vi "Production_of_Baker'sYeast_Repetitive_Fed_batch.vi"() -> ()   [LabVIEW 2019]
uses:
  <vilib>/addons/control/pid/pid.llb/PID Advanced (DBL).vi
  <vilib>/addons/control/pid/NI_PID_pid.lvlib
panel:
  out "Glucose Pipe 2":bool
  in  "process parameters":T1={"static gain"=2.5, "lag (s)"=2.5, "deadtime (s)"=0.001, "load"=0.0, "deadband"=0.0, "sensor noise"=0.0, "initial PV"=30.0, "plant noise"=0.0} {"plant noise" format="%.2f"; "initial PV" format="%.2f"; "sensor noise" format="%.2f"; "lag (s)" format="%.2f"; "deadtime (s)" format="%.2f"; "deadband" format="%.1f"; "load" format="%.2f"; "static gain" format="%.2f"}
  in  "SP Glucose 2":dbl(slide) scale=0.0..10.0
  in  "SP":dbl(knob) scale=0.0..100.0
  in  "auto? (T) 2":bool=TRUE
  in  "PID gains 2":T2={"proportional gain (Kc)"=1.0, "integral time (Ti, min)"=0.01, "derivative time (Td, min)"=0.0} {"derivative time (Td, min)" format="%.3f"; "integral time (Ti, min)" format="%.3f"; "proportional gain (Kc)" format="%.3f"}
  in  "LCV 2":dbl format="%.2f"
  out "Waveform Chart 2":T3(graph)
  out "Thermometer":dbl(slide) scale=0.0..100.0
  in  "process parameters 2":T1={"static gain"=2.5, "lag (s)"=2.5, "deadtime (s)"=0.001, "load"=0.0, "deadband"=0.0, "sensor noise"=0.0, "initial PV"=30.0, "plant noise"=0.0} {"plant noise" format="%.2f"; "initial PV" format="%.2f"; "sensor noise" format="%.2f"; "lag (s)" format="%.2f"; "deadtime (s)" format="%.2f"; "deadband" format="%.1f"; "load" format="%.2f"; "static gain" format="%.2f"}
  in  "LCV":dbl format="%.2f"
  in  "auto? (T)":bool=TRUE
  in  "SP Glucose":dbl(slide) scale=0.0..10.0
  in  "PID gains":T2={"proportional gain (Kc)"=1.0, "integral time (Ti, min)"=0.01, "derivative time (Td, min)"=0.0} {"derivative time (Td, min)" format="%.3f"; "integral time (Ti, min)" format="%.3f"; "proportional gain (Kc)" format="%.3f"}
  out "Waveform Chart":cluster{"output":dbl, dbl, "Plant Output":dbl}(graph)
  out "Multi-Segment Pipe":bool(c317)
  out "Storage":i32(slide) scale=0.0..450.0
  out "GLUCOSE":dbl(slide) scale=0.0..100.0
  out "Yeast bool":bool
  out "Yeast Pipe":bool
  out "YEAST (saccharomyces cerevisiae)":dbl(slide) scale=0.0..100.0
  out "Gauge":dbl(knob) scale=0.0..100.0 scale format="%#_3g"
  out "MIddle  bool":bool
  out "middle pipe":bool
  out "reactor bool":bool
  out "Glucose bool":bool
  out "Glucose Pipe":bool
  out "Mixtures":i32(slide) scale=0.0..250.0
  # "LCV"
  # "LT"
  # "REACTOR"
  # "CONTROL ROOM"
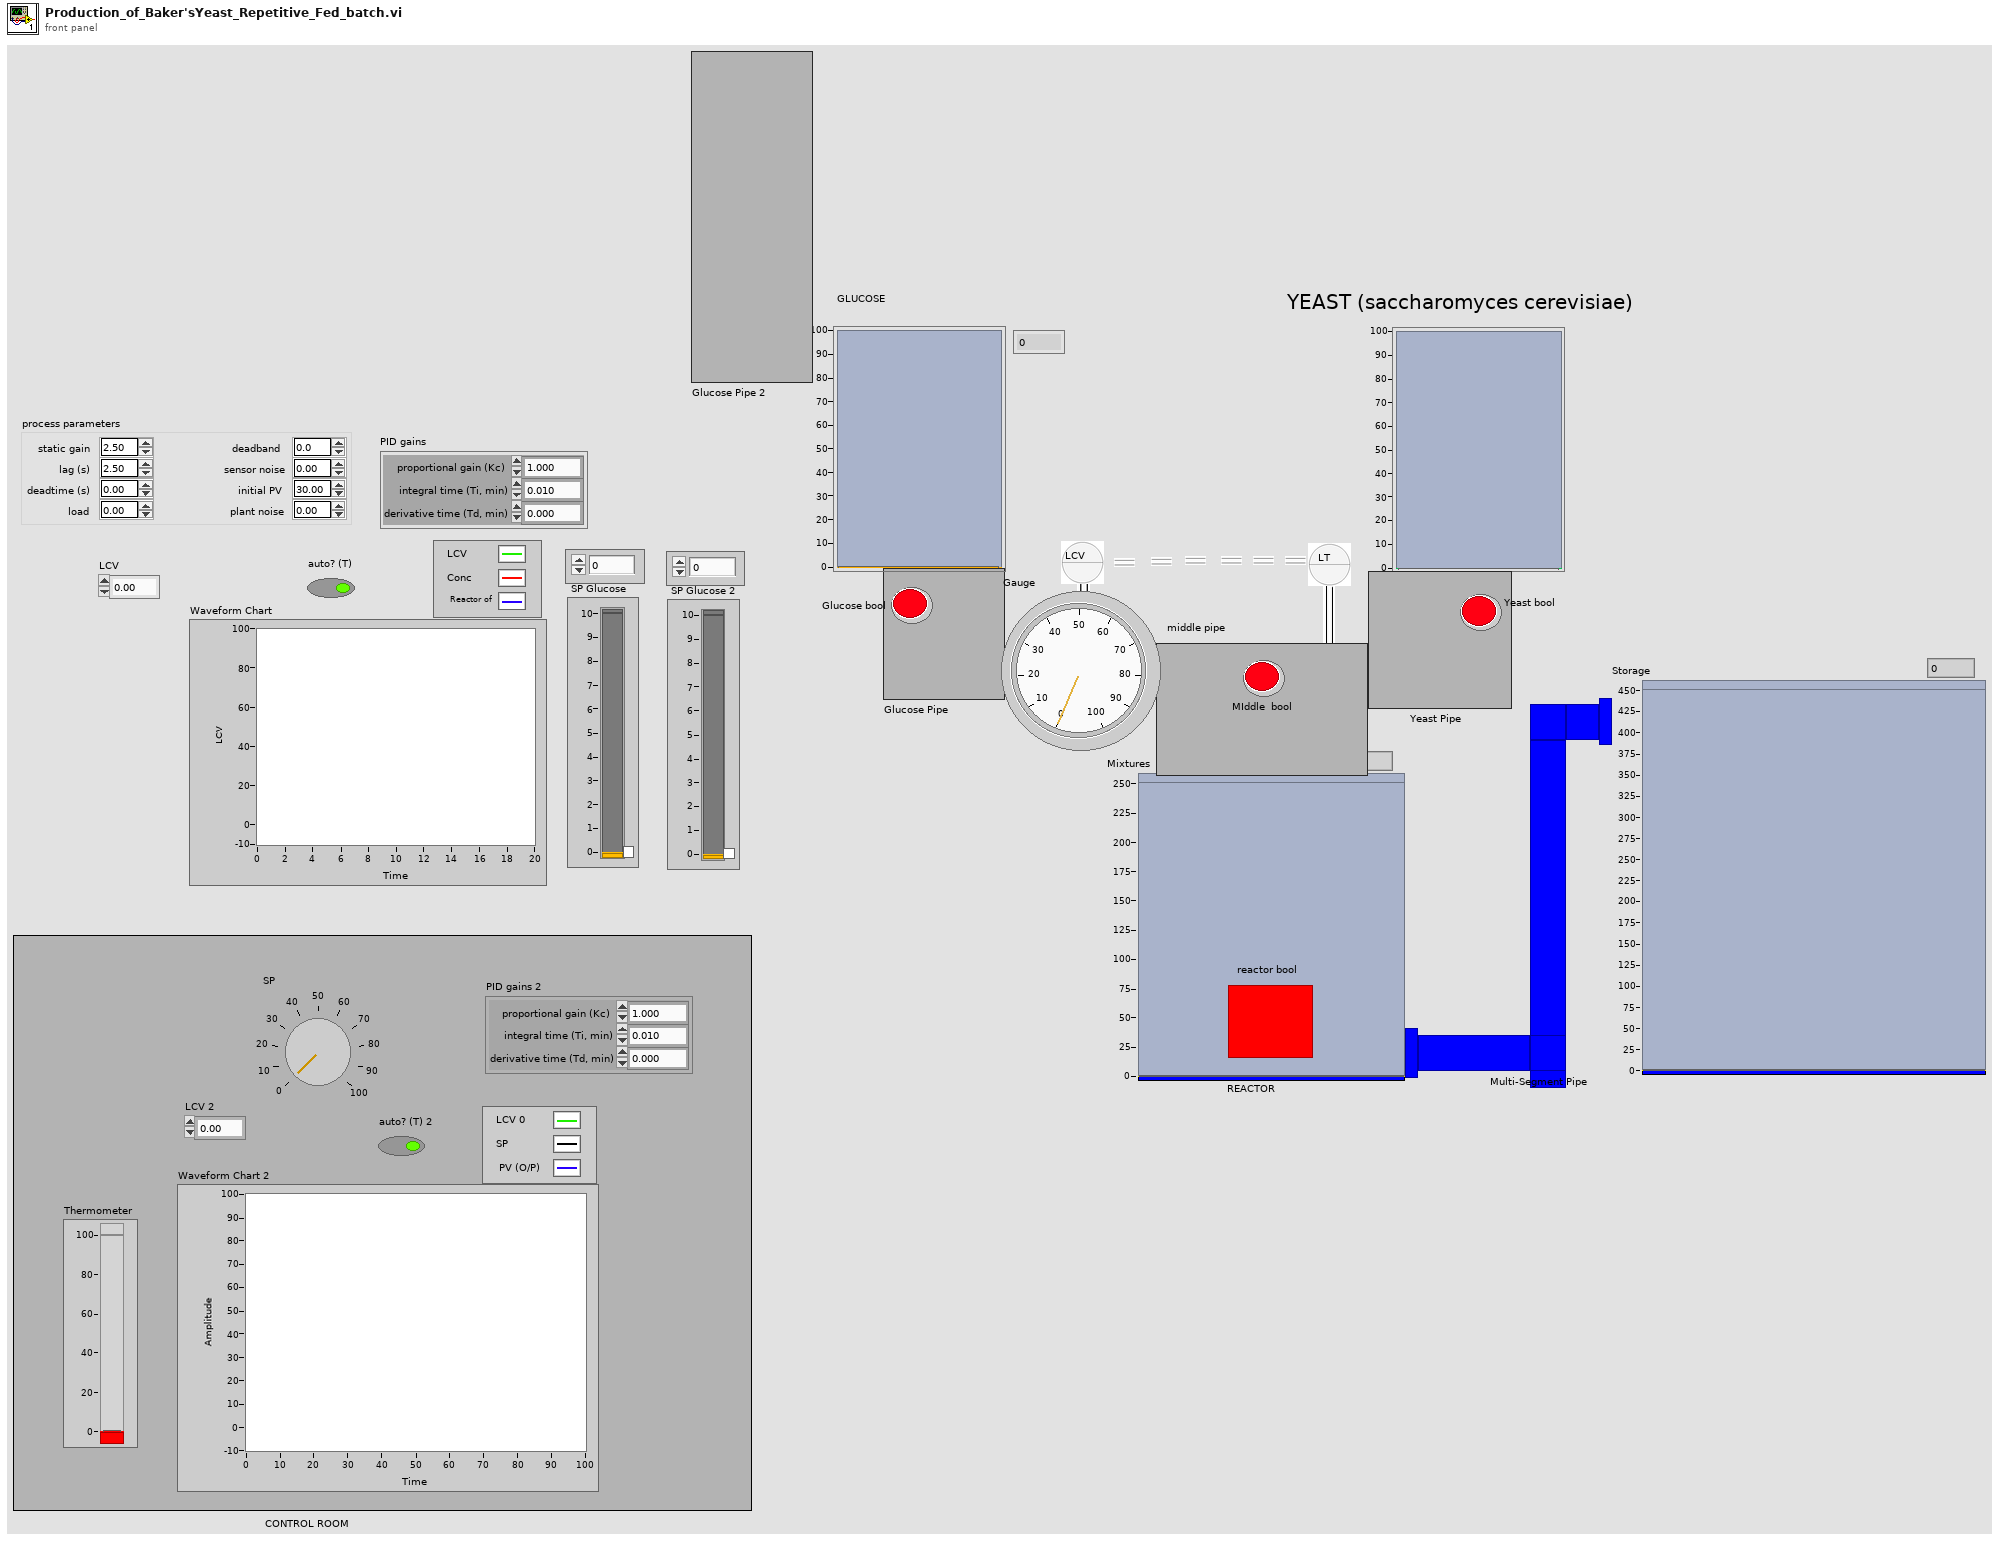
[diagram p1: front panel]
types:
  T1 = cluster{"static gain":dbl, "lag (s)":dbl, "deadtime (s)":dbl, "load":dbl, "deadband":dbl, "sensor noise":dbl, "initial PV":dbl, "plant noise":dbl}
  T2 = cluster{"proportional gain (Kc)":dbl, "integral time (Ti, min)":dbl, "derivative time (Td, min)":dbl}
  T3 = cluster{"LCV":dbl, " SP":dbl, "Plant Output":dbl}
  T4 = cluster{"output":dbl, "SP":dbl, "Plant Output":dbl}
diagram:
  n1 = flat-sequence {
    frame #0 {
      n2 = while {
        shift-right: [w17] -> _
        shift-left: 30.0 -> [w15]
        tunnel: TRUE ("Yeast bool") -> [w11]
        tunnel: FALSE ("Glucose bool") -> [w10]
        tunnel: FALSE ("reactor bool") -> [w9]
        tunnel: 0.0 ("Gauge") -> [w7]
        tunnel: 30.0 ("GLUCOSE") -> [w8]
        stop <- w13 stop-if-true
        n3 = property on="Storage" class="Slide (strict)"("Value"=w7) -> ()  [unwired: 2 in, 2 out]
        n4 = property on="Gauge" class="Knob (strict)"("Value"=w7) -> ()  [unwired: 2 in, 2 out]
        n5 = property on="GLUCOSE" class="Slide (strict)"("Value"=w8) -> ()  [unwired: 2 in, 2 out]
        n6 = property on="reactor bool" class="Bool (strict)"("Value"=w9) -> ()  [unwired: 2 in, 2 out]
        n7 = property on="MIddle  bool" class="Bool (strict)"("Value"=w11) -> ()  [unwired: 2 in, 2 out]
        n8 = property on="Glucose bool" class="Bool (strict)"("Value"=w10) -> ()  [unwired: 2 in, 2 out]
        n9 = Wait Until Next ms Multiple(millisecond multiple=u32 400) -> ()  [unwired: 1 out]
        n10 = property on="middle pipe" class="Bool (strict)"("Value"=w11) -> ()  [unwired: 2 in, 2 out]
        n11 = property on="Glucose Pipe" class="Bool (strict)"("Value"=w10) -> ()  [unwired: 2 in, 2 out]
        n12 = Subtract(x=30.0, y=w15) -> (x-y=w12:dbl)
        n13 = Equal?(x=w15, y=0.0) -> (x = y?=w13:bool)
        n14 = Decrement(x=w15) -> (x-1=w17:dbl)
        n15 = property on="Mixtures" class="Slide (strict)"("Value"=w12) -> ()  [unwired: 2 in, 2 out]
        "YEAST (saccharomyces cerevisiae)" <- w15
        "Yeast Pipe" <- w11
        "Yeast bool" <- w11
      }
    }
    frame #1 {
      n16 = while {
        border: 0.0 ("Plant Output") -> [_]
        tunnel: FALSE ("reactor bool") -> [w50]
        tunnel: TRUE ("Glucose bool") -> [w54]
        tunnel: TRUE ("MIddle  bool") -> [w53]
        stop <- w30 stop-if-true
        w38 = u32 100 ("millisecond multiple")
        w65 = u32 100 ("millisecond multiple")
        n17 = property on="Yeast bool" class="Bool (strict)"("Value"=w50) -> ()  [unwired: 2 in, 2 out]
        n18 = property on="reactor bool" class="Bool (strict)"("Value"=w50) -> ()  [unwired: 2 in, 2 out]
        n19 = property on="Yeast Pipe" class="Bool (strict)"("Value"=w50) -> ()  [unwired: 2 in, 2 out]
        n20 = Wait Until Next ms Multiple(millisecond multiple=w65) -> ()  [unwired: 1 out]
        n21 = Multiply(x=0.001, y=w65) -> (x*y=w40:dbl)
        n22 = Add(x="SP Glucose", y=30.0) -> (x+y=w49:dbl)
        n23 = Wait Until Next ms Multiple(millisecond multiple=w38) -> ()  [unwired: 1 out]
        n24 = Multiply(x=0.001, y=w38) -> (x*y=w36:dbl)
        n25 = property on="SP Glucose" class="Slide (strict)"() -> ("Value"=w26:dbl)  [unwired: 2 in, 2 out]
        n26 = Subtract(x=30.0 ("y"), y=w26) -> (x-y=w45:dbl)
        n27 = Wait Until Next ms Multiple(millisecond multiple=u32 600) -> ()  [unwired: 1 out]
        n28 = feedback #1() -> (w64:dbl)
        n29 = call-poly <vilib>:"PID Advanced.vi"("setpoint"=w49, "output range"=cluster{"output high":dbl, "output low":dbl} {"output high"=100.0, "output low"=0.0}, "auto? (T)"="auto? (T)", "manual control"="LCV", "process variable"=w64, "PID gains"="PID gains", "dt (s)"=w40) -> ("output"=w47:dbl)  [unwired: 7 in, 1 out]
        "Gauge" <- w47
        n30 = feedback #2() -> (w35:dbl)  [unwired: 1 in]
        n31 = call-poly <vilib>:"PID Advanced.vi"("setpoint"=w45, "output range"=cluster{"output high":dbl, "output low":dbl} {"output high"=100.0, "output low"=0.0}, "auto? (T)"="auto? (T)", "manual control"="LCV", "process variable"=w35, "PID gains"="PID gains", "dt (s)"=w36) -> ("output"=w24:dbl)  [unwired: 7 in, 1 out]
        n32 = property on="process parameters" class="Clust (strict)"() -> ("Value"=w23:T1)  [unwired: 2 in, 2 out]
        n33 = call "Plant System.vi"("output saturation range"=cluster{"output high":dbl, "output low":dbl} {"output high"=100.0, "output low"=0.0}, "Plant Input"=w47, "dt (s)"=w40, "process parameters"=w23) -> ("Plant Output"=w46:dbl)  [unwired: 11 in]
        n34 = feedback-in #1(w46) -> ()
        n35 = call "Plant System.vi"("output saturation range"=cluster{"output high":dbl, "output low":dbl} {"output high"=100.0, "output low"=0.0}, "Plant Input"=w24, "dt (s)"=w36, "process parameters"=w23) -> ("Plant Output"=w34:dbl)  [unwired: 11 in]
        "GLUCOSE" <- w34
        n36 = feedback-in #2(w34) -> ()
        n37 = property on="SP Glucose" class="Slide (strict)"() -> ("Value"=w59:dbl)  [unwired: 2 in, 2 out]
        n38 = property on="SP Glucose" class="Slide (strict)"() -> ("Value"=w29:dbl)  [unwired: 2 in, 2 out]
        n39 = Bundle("output"=w47, w49, "Plant Output"=w46) -> (→"Waveform Chart":cluster{"output":dbl, dbl, "Plant Output":dbl})  [unwired: 1 in]
        n40 = Add(x=30.0, y=w59) -> (x+y=w58:dbl)
        n41 = property on="Mixtures" class="Slide (strict)"() -> ("Value"=w52:i32)  [unwired: 2 in, 2 out]
        n42 = property on="GLUCOSE" class="Slide (strict)"() -> ("Value"=w33:dbl)  [unwired: 2 in, 2 out]
        n43 = Subtract(x=30.0, y=w29) -> (x-y=w25:dbl)
        n44 = Add(x=w46, y=0.0) -> (x+y=→"Mixtures":dbl)
        n45 = Greater Or Equal?(x=w52, y=w58) -> (x >= y?=w32:bool)
        n46 = Less Or Equal?(x=w33, y=w25) -> (x <= y?=w31:bool)
        n47 = And(x=w32, y=w31) -> (x .and. y?=w30:bool)
        "Glucose bool" <- w54
        "Glucose Pipe" <- w54
        "MIddle  bool" <- w53
        "middle pipe" <- w53
      }
    }
    frame #2 {
      n48 = while {
        stop <- w67 stop-if-true
        w80 = u32 100 ("millisecond multiple")
        n49 = Wait Until Next ms Multiple(millisecond multiple=w80) -> ()  [unwired: 1 out]
        n50 = Multiply(x=0.001, y=w80) -> (x*y=w78:dbl)
        n51 = property on="Thermometer" class="Slide (strict)"() -> ("Value"=w70:dbl)  [unwired: 2 in, 2 out]
        n52 = call-poly <vilib>:"PID Advanced.vi"("setpoint"="SP", "output range"=cluster{"output high":dbl, "output low":dbl} {"output high"=100.0, "output low"=0.0}, "auto? (T)"="auto? (T) 2", "manual control"="LCV 2", "process variable"=w70, "PID gains"="PID gains 2", "dt (s)"=w78) -> ("output"=w74:dbl)  [unwired: 7 in, 1 out]
        n53 = call "Plant System.vi"("output saturation range"=cluster{"output high":dbl, "output low":dbl} {"output high"=100.0, "output low"=0.0}, "Plant Input"=w74, "dt (s)"=w78, "process parameters"="process parameters 2") -> ("Plant Output"=w72:dbl)  [unwired: 11 in]
        "Thermometer" <- w72
        n54 = Bundle("output"=w74, "SP"="SP", "Plant Output"=w72) -> (→"Waveform Chart 2":T4)  [unwired: 1 in]
        n55 = property on="Thermometer" class="Slide (strict)"() -> ("Value"=w69:dbl)  [unwired: 2 in, 2 out]
        n56 = property on="SP" class="Knob (strict)"() -> ("Value"=w68:dbl)  [unwired: 2 in, 2 out]
        n57 = Greater Or Equal?(x=w69, y=w68) -> (x >= y?=w67:bool)
      }
    }
    frame #3 {
      n58 = property on="Mixtures" class="Slide (strict)"() -> ("Value"=w85:i32)  [unwired: 2 in, 2 out]
      n59 = while {
        shift-right: [w93] -> _
        shift-left: w85 -> [w94]
        tunnel: TRUE ("reactor bool") -> [w92]
        stop <- w95 stop-if-true
        n60 = property on="SP Glucose" class="Slide (strict)"() -> ("Value"=w87:dbl)  [unwired: 2 in, 2 out]
        n61 = Add(x=30.0, y=w87) -> (x+y=w86:dbl)
        n62 = property on="Mixtures" class="Slide (strict)"("Value"=w94) -> ()  [unwired: 2 in, 2 out]
        n63 = Scale By Power Of 2(n=i16 2, x=w86) -> (x*2^n=w89:dbl)
        n64 = Increment(x=w94) -> (x+1=w93:i32)
        n65 = Greater Or Equal?(x=w93, y=w89) -> (x >= y?=w95:bool)
        n66 = Wait Until Next ms Multiple(millisecond multiple=u32 1000) -> ()  [unwired: 1 out]
        "reactor bool" <- w92
      }
    }
    frame #4 {
      n67 = property on="Mixtures" class="Slide (strict)"() -> ("Value"=w97:i32)  [unwired: 2 in, 2 out]
      n68 = while {
        shift-right: [w110] -> _
        shift-left: w97 -> [w106]
        tunnel: TRUE ("Multi-Segment Pipe") -> [w104]
        stop <- w108 stop-if-true
        n69 = property on="SP Glucose" class="Slide (strict)"() -> ("Value"=w99:dbl)  [unwired: 2 in, 2 out]
        n70 = Wait Until Next ms Multiple(millisecond multiple=u32 400) -> ()  [unwired: 1 out]
        n71 = Add(x=30.0, y=w99) -> (x+y=w98:dbl)
        n72 = property on="Mixtures" class="Slide (strict)"("Value"=w106) -> ()  [unwired: 2 in, 2 out]
        n73 = Scale By Power Of 2(n=i16 2, x=w98) -> (x*2^n=w102:dbl)
        n74 = Add(x=0.0, y=w102) -> (x+y=w105:dbl)
        n75 = Equal?(x=w106, y=30.0) -> (x = y?=w108:bool)
        n76 = Subtract(x=w105, y=w106) -> (x-y=→"Storage":dbl)
        n77 = Decrement(x=w106) -> (x-1=w110:i32)
        "Multi-Segment Pipe" <- w104
      }
    }
    frame #5 {
      n78 = property on="GLUCOSE" class="Slide (strict)"() -> ("Value"=w114:dbl)  [unwired: 2 in, 2 out]
      n79 = while {
        shift-right: [w120] -> _
        shift-left: w114 -> [w118]
        tunnel: TRUE ("Glucose Pipe 2") -> [w116]
        tunnel: TRUE ("reactor bool") -> [w115]
        stop <- w121 stop-if-true
        n80 = property on="reactor bool" class="Bool (strict)"("Value"=w115) -> ()  [unwired: 2 in, 2 out]
        n81 = property on="GLUCOSE" class="Slide (strict)"("Value"=w118) -> ()  [unwired: 2 in, 2 out]
        n82 = Increment(x=w118) -> (x+1=w120:dbl)
        n83 = Greater Or Equal?(x=w120, y=30.0) -> (x >= y?=w121:bool)
        n84 = Wait Until Next ms Multiple(millisecond multiple=u32 1000) -> ()  [unwired: 1 out]
        "Glucose Pipe 2" <- w116
      }
    }
    frame #6 {
      n85 = while {
        border: 0.0 ("Plant Output") -> [_]
        tunnel: FALSE ("reactor bool") -> [w127]
        tunnel: TRUE ("Glucose bool") -> [w134]
        tunnel: TRUE ("MIddle  bool") -> [w126]
        stop <- w150 stop-if-true
        w156 = u32 100 ("millisecond multiple")
        w170 = u32 100 ("millisecond multiple")
        n86 = property on="reactor bool" class="Bool (strict)"("Value"=w126) -> ()  [unwired: 2 in, 2 out]
        n87 = property on="middle pipe" class="Bool (strict)"("Value"=w126) -> ()  [unwired: 2 in, 2 out]
        n88 = property on="Glucose Pipe" class="Bool (strict)"("Value"=w126) -> ()  [unwired: 2 in, 2 out]
        n89 = property on="Yeast bool" class="Bool (strict)"("Value"=w127) -> ()  [unwired: 2 in, 2 out]
        n90 = property on="MIddle  bool" class="Bool (strict)"("Value"=w134) -> ()  [unwired: 2 in, 2 out]
        n91 = property on="PID gains" class="Clust (strict)"() -> ("Value"=w146:T2)  [unwired: 2 in, 2 out]
        n92 = property on="Yeast Pipe" class="Bool (strict)"("Value"=w127) -> ()  [unwired: 2 in, 2 out]
        n93 = property on="Glucose bool" class="Bool (strict)"("Value"=w134) -> ()  [unwired: 2 in, 2 out]
        n94 = Wait Until Next ms Multiple(millisecond multiple=w170) -> ()  [unwired: 1 out]
        n95 = Multiply(x=0.001, y=w170) -> (x*y=w158:dbl)
        n96 = property on="SP Glucose 2" class="Slide (strict)"() -> ("Value"=w130:dbl)  [unwired: 2 in, 2 out]
        n97 = property on="LCV" class="DigNum (strict)"() -> ("Value"=w144:dbl)  [unwired: 2 in, 2 out]
        n98 = Add(x="SP Glucose 2", y=30.0) -> (x+y=w163:dbl)
        n99 = property on="auto? (T)" class="Bool (strict)"() -> ("Value"=w145:bool)  [unwired: 2 in, 2 out]
        n100 = Wait Until Next ms Multiple(millisecond multiple=w156) -> ()  [unwired: 1 out]
        n101 = Multiply(x=0.001, y=w156) -> (x*y=w154:dbl)
        n102 = Subtract(x=30.0, y=w130) -> (x-y=w132:dbl)
        n103 = Subtract(x=0.0, y=w132) -> (x-y=w160:dbl)
        n104 = Wait Until Next ms Multiple(millisecond multiple=u32 600) -> ()  [unwired: 1 out]
        n105 = feedback #3() -> (w169:dbl)
        n106 = call-poly <vilib>:"PID Advanced.vi"("setpoint"=w163, "output range"=cluster{"output high":dbl, "output low":dbl} {"output high"=100.0, "output low"=0.0}, "auto? (T)"=w145, "manual control"=w144, "process variable"=w169, "PID gains"=w146, "dt (s)"=w158) -> ("output"=w135:dbl)  [unwired: 7 in, 1 out]
        n107 = feedback #4() -> (w153:dbl)  [unwired: 1 in]
        n108 = call-poly <vilib>:"PID Advanced.vi"("setpoint"=w160, "output range"=cluster{"output high":dbl, "output low":dbl} {"output high"=100.0, "output low"=0.0}, "auto? (T)"=w145, "manual control"=w144, "process variable"=w153, "PID gains"=w146, "dt (s)"=w154) -> ("output"=w147:dbl)  [unwired: 7 in, 1 out]
        n109 = call "Plant System.vi"("output saturation range"=cluster{"output high":dbl, "output low":dbl} {"output high"=100.0, "output low"=0.0}, "Plant Input"=w135, "dt (s)"=w158, "process parameters"="process parameters") -> ("Plant Output"=w161:dbl)  [unwired: 11 in]
        n110 = feedback-in #3(w161) -> ()
        n111 = call "Plant System.vi"("output saturation range"=cluster{"output high":dbl, "output low":dbl} {"output high"=100.0, "output low"=0.0}, "Plant Input"=w147, "dt (s)"=w154, "process parameters"="process parameters") -> ("Plant Output"=w136:dbl)  [unwired: 11 in]
        n112 = feedback-in #4(w136) -> ()
        n113 = property on="Gauge" class="Knob (strict)"("Value"=w135) -> ()  [unwired: 2 in, 2 out]
        n114 = property on="SP Glucose 2" class="Slide (strict)"() -> ("Value"=w139:dbl)  [unwired: 2 in, 2 out]
        n115 = property on="SP Glucose 2" class="Slide (strict)"() -> ("Value"=w137:dbl)  [unwired: 2 in, 2 out]
        n116 = Bundle("output"=w135, w163, "Plant Output"=w161) -> (w142:cluster{"output":dbl, dbl, "Plant Output":dbl})  [unwired: 1 in]
        n117 = property on="Mixtures" class="Slide (strict)"() -> ("Value"=w138:i32)  [unwired: 2 in, 2 out]
        n118 = property on="GLUCOSE" class="Slide (strict)"() -> ("Value"=w143:dbl)  [unwired: 2 in, 2 out]
        n119 = Add(x=30.0, y=w139) -> (x+y=w166:dbl)
        n120 = Subtract(x=30.0, y=w137) -> (x-y=w148:dbl)
        n121 = Add(x=w161, y=0.0) -> (x+y=w141:dbl)
        n122 = Greater Or Equal?(x=w138, y=w166) -> (x >= y?=w152:bool)
        n123 = Less Or Equal?(x=w143, y=w148) -> (x <= y?=w151:bool)
        n124 = property on="Waveform Chart" class="WFChart (strict)"("Value"=w142) -> ()  [unwired: 2 in, 2 out]
        n125 = And(x=w152, y=w151) -> (x .and. y?=w150:bool)
        n126 = property on="Mixtures" class="Slide (strict)"("Value"=w141) -> ()  [unwired: 2 in, 2 out]
        n127 = property on="GLUCOSE" class="Slide (strict)"("Value"=w136) -> ()  [unwired: 2 in, 2 out]
      }
    }
    frame #7 {
      n128 = property on="Mixtures" class="Slide (strict)"() -> ("Value"=w174:i32)  [unwired: 2 in, 2 out]
      n129 = while {
        shift-right: [w184] -> _
        shift-left: w174 -> [w178]
        tunnel: TRUE ("reactor bool") -> [w176]
        tunnel: FALSE ("Glucose bool") -> [w175]
        stop <- w185 stop-if-true
        n130 = property on="SP Glucose 2" class="Slide (strict)"() -> ("Value"=w177:dbl)  [unwired: 2 in, 2 out]
        n131 = property on="Glucose bool" class="Bool (strict)"("Value"=w175) -> ()  [unwired: 2 in, 2 out]
        n132 = property on="reactor bool" class="Bool (strict)"("Value"=w176) -> ()  [unwired: 2 in, 2 out]
        n133 = Add(x=30.0, y=w177) -> (x+y=w179:dbl)
        n134 = property on="Mixtures" class="Slide (strict)"("Value"=w178) -> ()  [unwired: 2 in, 2 out]
        n135 = Scale By Power Of 2(n=i16 2, x=w179) -> (x*2^n=w181:dbl)
        n136 = property on="MIddle  bool" class="Bool (strict)"("Value"=w175) -> ()  [unwired: 2 in, 2 out]
        n137 = property on="Glucose Pipe" class="Bool (strict)"("Value"=w175) -> ()  [unwired: 2 in, 2 out]
        n138 = property on="middle pipe" class="Bool (strict)"("Value"=w175) -> ()  [unwired: 2 in, 2 out]
        n139 = Increment(x=w178) -> (x+1=w184:i32)
        n140 = Greater Or Equal?(x=w184, y=w181) -> (x >= y?=w185:bool)
        n141 = Wait Until Next ms Multiple(millisecond multiple=u32 1000) -> ()  [unwired: 1 out]
      }
    }
    frame #8 {
      n142 = property on="Mixtures" class="Slide (strict)"() -> ("Value"=w187:i32)  [unwired: 2 in, 2 out]
      n143 = while {
        shift-right: [w204] -> _
        shift-left: w187 -> [w196]
        tunnel: TRUE ("Multi-Segment Pipe") -> [w194]
        stop <- w202 stop-if-true
        n144 = property on="SP Glucose 2" class="Slide (strict)"() -> ("Value"=w195:dbl)  [unwired: 2 in, 2 out]
        n145 = property on="Multi-Segment Pipe" class="MultiSegPipe"("Value"=w194) -> ()  [unwired: 2 in, 2 out]
        n146 = Add(x=30.0, y=w195) -> (x+y=w193:dbl)
        n147 = Wait Until Next ms Multiple(millisecond multiple=u32 400) -> ()  [unwired: 1 out]
        n148 = Add(x=w193, y=0.0) -> (x+y=w192:dbl)
        n149 = property on="Mixtures" class="Slide (strict)"("Value"=w196) -> ()  [unwired: 2 in, 2 out]
        n150 = Scale By Power Of 2(n=i16 2, x=w192) -> (x*2^n=w199:dbl)
        n151 = Add(x=0.0, y=w199) -> (x+y=w201:dbl)
        n152 = Equal?(x=w196, y=0.0) -> (x = y?=w202:bool)
        n153 = Subtract(x=w201, y=w196) -> (x-y=w190:dbl)
        n154 = Decrement(x=w196) -> (x-1=w204:i32)
        n155 = Add(x=w190, y=110.0) -> (x+y=w191:dbl)
        n156 = property on="Storage" class="Slide (strict)"("Value"=w191) -> ()  [unwired: 2 in, 2 out]
      }
    }
  }
